vi "ExtractHarmonics.vi"(8 "highest harmonic":i32=19, 11 "Input cluster":T1) -> (2 "components level":dbl[](array[numeric]) format="%.2p", 3 "detected fundamental frequency":dbl format="%.2p")   [LabVIEW 2019]
uses:
  <vilib>/measure/matone.llb/Harmonic Distortion Analyzer 1 Chan.vi
  <vilib>/measure/NI_MAPro.lvlib
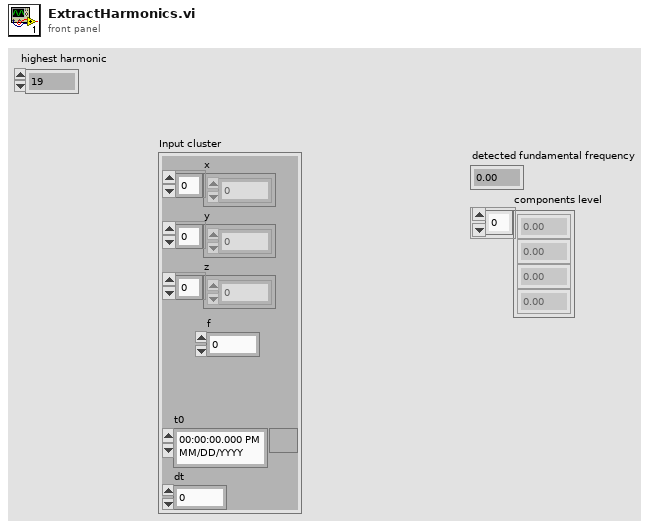
[diagram p1: front panel]
types:
  T1 = cluster{"x":dbl[], "y":dbl[], "z":dbl[], "t0":timestamp, "dt":dbl, "f":dbl}
  T2 = cluster{"approx freq. (optional)":dbl, "search (+/- % of Fsampl.)":dbl}
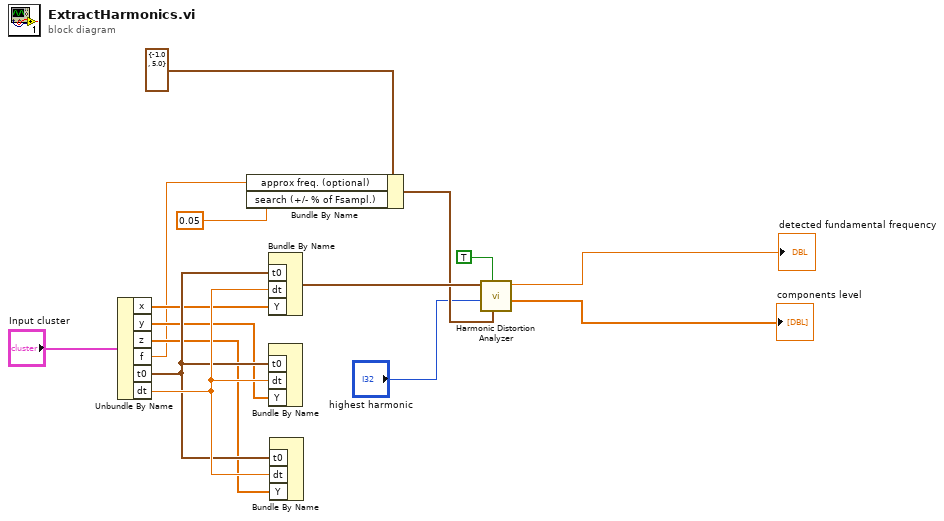
[diagram p0: block diagram]
diagram:
  n1 = Unbundle By Name("Input cluster") -> ("x"=w12:dbl[], "y"=w11:dbl[], "z"=w10:dbl[], "f"=w1:dbl, "t0"=w13:timestamp, "dt"=w14:dbl)
  n2 = Bundle By Name(cluster=T2 {"approx freq. (optional)"=-1.0, "search (+/- % of Fsampl.)"=5.0} ("advanced search"), "approx freq. (optional)"=w1, "search (+/- % of Fsampl.)"=0.05) -> (w6:T2)
  n3 = Bundle By Name("t0"=w13, "dt"=w14, "Y"=w12) -> (w9:waveform(dbl))  [unwired: 1 in]
  n4 = Bundle By Name("t0"=w13, "dt"=w14, "Y"=w11) -> ()  [unwired: 1 in, 1 out]
  n5 = Bundle By Name("t0"=w13, "dt"=w14, "Y"=w10) -> ()  [unwired: 1 in, 1 out]
  n6 = call-poly <vilib>:"Harmonic Distortion Analyzer.vi"("advanced search"=w6, "stop search at Nyquist"=TRUE, "highest harmonic"="highest harmonic", "signal in"=w9) -> ("components level"=→"components level":dbl[], "detected fundamental frequency"=→"detected fundamental frequency":dbl)  [unwired: 2 in, 4 out]
